vi "Set Stop.vi"(7 "Server Alias":string, 10 "Error In":errorcluster, 11 "Stop":bool) -> (2 "Error Out":errorcluster)   [LabVIEW 2013, in "TS.lvlib"]
uses:
  TS.lvlib
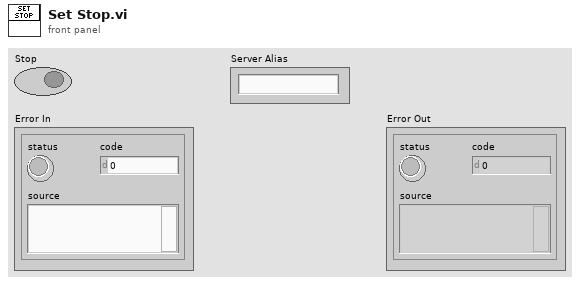
[diagram p1: front panel]
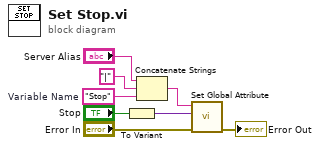
[diagram p0: block diagram]
diagram:
  w5 = "Stop"  # Variable Name
  n1 = To Variant(anything="Stop") -> (Variant=w1:variant)
  n2 = Concatenate Strings("Server Alias", "|" ("string"), w5) -> (w4:string)
  n3 = call "Set Global Attribute.vi"("Error In"="Error In", "Value"=w1, "Name"=w4) -> ("Error Out"=→"Error Out":errorcluster)  [unwired: 7 in, 1 out]
